vi "SetParam.vi"(8 "error in (no error)":errorcluster caption="entrée d'erreur (pas d'erreur)", 10 "normalized_mutual_info_score":cluster{"average_method":string}={"average_method"="arithmetic"}, 11 "Normalized_Mutual_Info_Score.lvclass":refnum<class "Normalized_Mutual_Info_Score.lvclass">) -> (0 "error out":errorcluster caption="sortie d'erreur", 3 "Normalized_Mutual_Info_Score.lvclass":refnum<class "Normalized_Mutual_Info_Score.lvclass">)   [LabVIEW 2020, in "Normalized_Mutual_Info_Score.lvclass"]
doc: "Set Parameters"
uses:
  Normalized_Mutual_Info_Score.lvclass
  Normalized_Mutual_Info_Score.lvclass/Normalized_Mutual_Info_Score.ctl
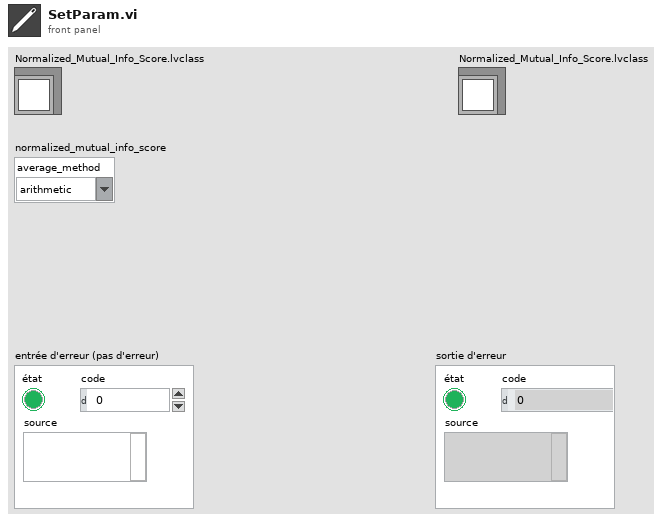
[diagram p1: front panel]
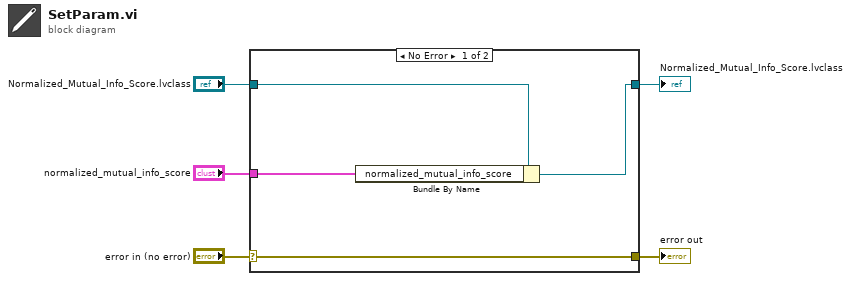
[diagram p0: block diagram]
diagram:
  n1 = case shown="No Error" "error in (no error)" {
    selector: "error in (no error)" -> [w9 w10]
    tunnel: [w9 w10] -> w4
    tunnel: [w7 w11] -> w2
    tunnel: "Normalized_Mutual_Info_Score.lvclass" -> [w8 w11]
    tunnel: "normalized_mutual_info_score" -> [w6 _]
    frame No Error {
      n2 = Bundle By Name(cluster=w8, "normalized_mutual_info_score"=w6) -> (w7:refnum<class "Normalized_Mutual_Info_Score.lvclass">)
    }
    frame Error {
    }
  }
  "error out" <- w4
  "Normalized_Mutual_Info_Score.lvclass" <- w2
